vi "停止发送CAN.vi"(8 "错误输入":errorcluster caption="错误常量") -> (0 "错误输出":errorcluster caption="错误常量")   [LabVIEW 2020]
uses:
  Global_Variable/Global.vi
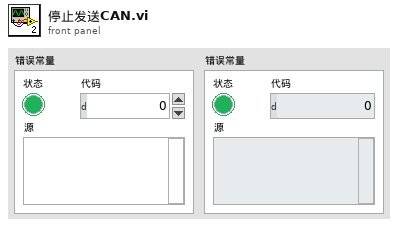
[diagram p1: front panel]
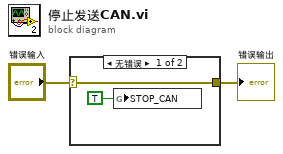
[diagram p0: block diagram]
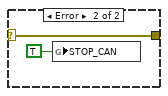
[diagram p2: hidden frame]
diagram:
  n1 = case shown="无错误" "错误输入" {
    selector: "错误输入" -> [w3 w6]
    tunnel: [w3 w6] -> w1
    frame No Error {
      n2 = global write "Global.vi" "STOP_CAN"(TRUE ("STOP_CAN")) -> ()
    }
    frame Error {
      n3 = global write "Global.vi" "STOP_CAN"(TRUE ("STOP_CAN")) -> ()
    }
  }
  "错误输出" <- w1
